vi "Node - Reader.vi"(8 "error in (no error)":errorcluster, 11 "Node Data In":T1) -> (0 "error out":errorcluster, 3 "Node Data Out":T1)   [LabVIEW 2016, in "PXImc Router.lvlib"]
uses:
  PXImc Router.lvlib
  Controls/Node Data.ctl
  <vilib>/NI Veristand/VeriStand Data/Byte Buffer/Byte Buffer.lvclass
  Controls/Node/Node - PXImc Parameters.ctl
  Controls/Node/Node - Writer Data.ctl
  Controls/Node/Node Ch Properties.ctl
  Controls/Data Type.ctl
  Controls/Node/Node - Readers Data.ctl
  Controls/Node/Node - Reader Data.ctl
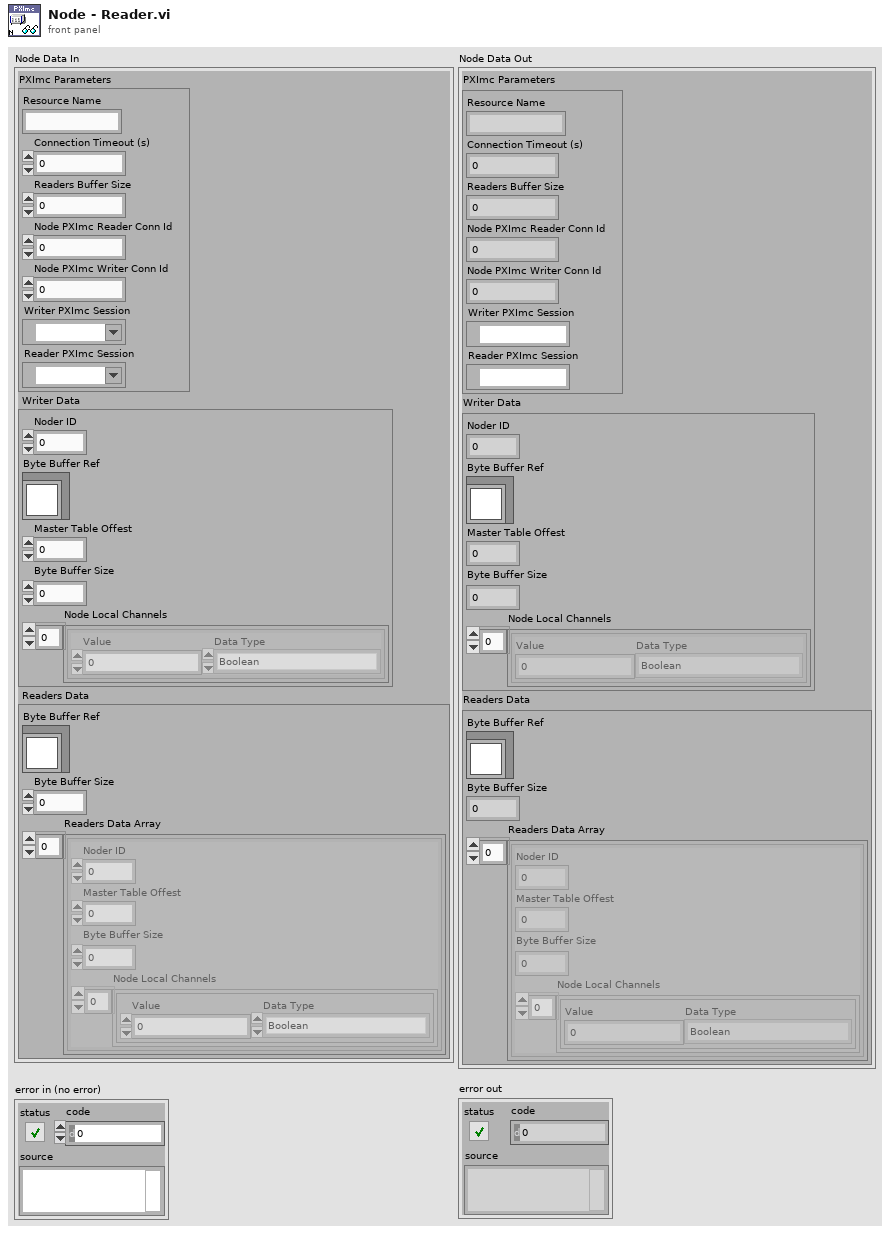
[diagram p1: front panel]
types:
  T1 = typedef "PXImc Router.lvlib/Node Data.ctl" = cluster{"PXImc Parameters":T2, "Writer Data":T3, "Readers Data":T6}
  T2 = typedef "PXImc Router.lvlib/Node - PXImc Parameters.ctl" = cluster{"Resource Name":string, "Connection Timeout (s)":dbl, "Readers Buffer Size":u64, "Node PXImc Reader Conn Id":u16, "Node PXImc Writer Conn Id":u16, "Writer PXImc Session":refnum<k21>, "Reader PXImc Session":refnum<k21>}
  T3 = typedef "PXImc Router.lvlib/Node - Writer Data.ctl" = cluster{"Noder ID":u32, "Byte Buffer Ref":refnum<class "Byte Buffer.lvclass">, "Master Table Offest":u32, "Byte Buffer Size":u32, "Node Local Channels":T4[]}
  T4 = typedef "PXImc Router.lvlib/Node Ch Properties.ctl" = cluster{"Value":dbl, "Data Type":T5}
  T5 = typedef "PXImc Router.lvlib/Data Type.ctl" = enum16{"Boolean", "SGL", "DBL", "I8", "I16", "I32", "I64", "U8", "U16", "U32", "U64"}
  T6 = typedef "PXImc Router.lvlib/Node - Readers Data.ctl" = cluster{"Byte Buffer Ref":refnum<class "Byte Buffer.lvclass">, "Byte Buffer Size":u64, "Readers Data Array":T7[]}
  T7 = typedef "PXImc Router.lvlib/Node - Reader Data.ctl" = cluster{"Noder ID":u32, "Master Table Offest":u32, "Byte Buffer Size":u64, "Node Local Channels":T4[]}
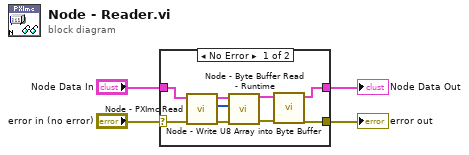
[diagram p0: block diagram]
diagram:
  n1 = case shown="No Error" "error in (no error)" {
    selector: "error in (no error)" -> [w12 w14]
    tunnel: [w6 w14] -> w4
    tunnel: "Node Data In" -> [w13 w15]
    tunnel: [w7 w15] -> w2
    frame No Error {
      n2 = call "Node - PXImc Read.vi"("error in (no error)"=w12, "Node Data In"=w13) -> ("error out"=w11:errorcluster, "Readers Data Out"=w5:u8[], "Node Data In"=w10:T1)  [unwired: 7 in]
      n3 = call "Node - Write U8 Array into Byte Buffer.vi"("error in (no error)"=w11, "U8 Array In"=w5, "Node Data In"=w10) -> ("error out"=w8:errorcluster, "Node Data Out"=w9:T1)  [unwired: 7 in]
      n4 = call "Node - Byte Buffer Read - Runtime.vi"("error in (no error)"=w8, "Node Data In"=w9) -> ("error out"=w6:errorcluster, "Node Data Out"=w7:T1)  [unwired: 7 in, 1 out]
    }
    frame Error {
    }
  }
  "error out" <- w4
  "Node Data Out" <- w2
